vi "AuMT8852B Multiple-slot Sensitivity Configuration.vi"(5 "Settings":T1={"Low frequency selection"=enum."Use low frequency", "Medium frequency selection"=enum."Use medium frequency", "High frequency selection"=enum."Use high frequency", "Low TX frequency"=2480.0, "Low RX frequency"=2402.0, "Medium TX frequency"=2402.0, "Medium RX frequency"=2441.0, "High TX frequency"=2402.0, "High RX frequency"=2480.0, "Number of packets"=590, "TX power"=-70.0, "BER limit"=0.1, "FER limit"=100.0, "Hop selection"=enum."Test with hopping off and on", "Packet type"=enum."Longest supported", "Use Dirty transmitter"=TRUE, "Frequency offset (kHz)"=[71.0, 14.0, -2.0, 1.0, 39.0, 0.0, -42.0, 74.0, -19.0, -75.0], "Modulation index"=[0.33, 0.3, 0.29, 0.32, 0.33, 0.34, 0.29, 0.31, 0.28, 0.35], "Symbol timing error (ppm)"=[-20.0, 20.0, 20.0, 20.0, 20.0, -20.0, -20.0, -20.0, -20.0, 20.0], "Packet count"=enum."RX"} {"Symbol timing error (ppm)" format="%.2f"; "Modulation index" format="%.2f"; "Frequency offset (kHz)" format="%.2f"; "FER limit" format="%.2f"; "BER limit" format="%.2f"; "TX power" format="%.1f"}, 7 "Set/Get (Set)":enum16{"Set", "Get"}(ring), 8 "error in (no error)":errorcluster, 10 "Script (3)":i32=3, 11 "VISA session":refnum<visa-resource-name>) -> (0 "error out":errorcluster, 2 "error code":i32, 3 "VISA session out":refnum<visa-resource-name>, 4 "Settings out":T1={"Low frequency selection"=enum."Use low frequency", "Medium frequency selection"=enum."Use medium frequency", "High frequency selection"=enum."Use high frequency", "Low TX frequency"=0.0, "Low RX frequency"=0.0, "Medium TX frequency"=0.0, "Medium RX frequency"=0.0, "High TX frequency"=0.0, "High RX frequency"=0.0, "Number of packets"=0, "TX power"=0.0, "BER limit"=0.0, "FER limit"=0.0, "Hop selection"=enum."Test with hopping on", "Packet type"=enum."Longest supported", "Use Dirty transmitter"=FALSE, "Frequency offset (kHz)"=[], "Modulation index"=[], "Symbol timing error (ppm)"=[], "Packet count"=enum."TX"} {"Symbol timing error (ppm)" format="%.2f"; "Modulation index" format="%.2f"; "Frequency offset (kHz)" format="%.2f"; "FER limit" format="%.2f"; "BER limit" format="%.2f"; "TX power" format="%.1f"})   [LabVIEW 2017]
doc: "Anritsu MT8852B Bluetooth Tester\n\nConfigures the instrument for the Multiple-slot Sensitivity test.\n\nINPUTS\nSet/Get - whether the values are being sent to or retrieved from the instrument.\nScript - which of the stored scripts (1-10) will be queried or configured. Scripts 1 and 2 are read-only.\nSettings - parameters of the test to be written.\n\nOUTPUTS\nSettings out - current parameters of the test."
uses:
  <instrlib>/aumt8852B/General/Utilities/MT8850 Test Parameters.ctl
  <instrlib>/aumt8852B/General/Utilities/MT8850 Frequency Units.ctl
panel:
  in  "Case Constant\n(See Context Help)":bool
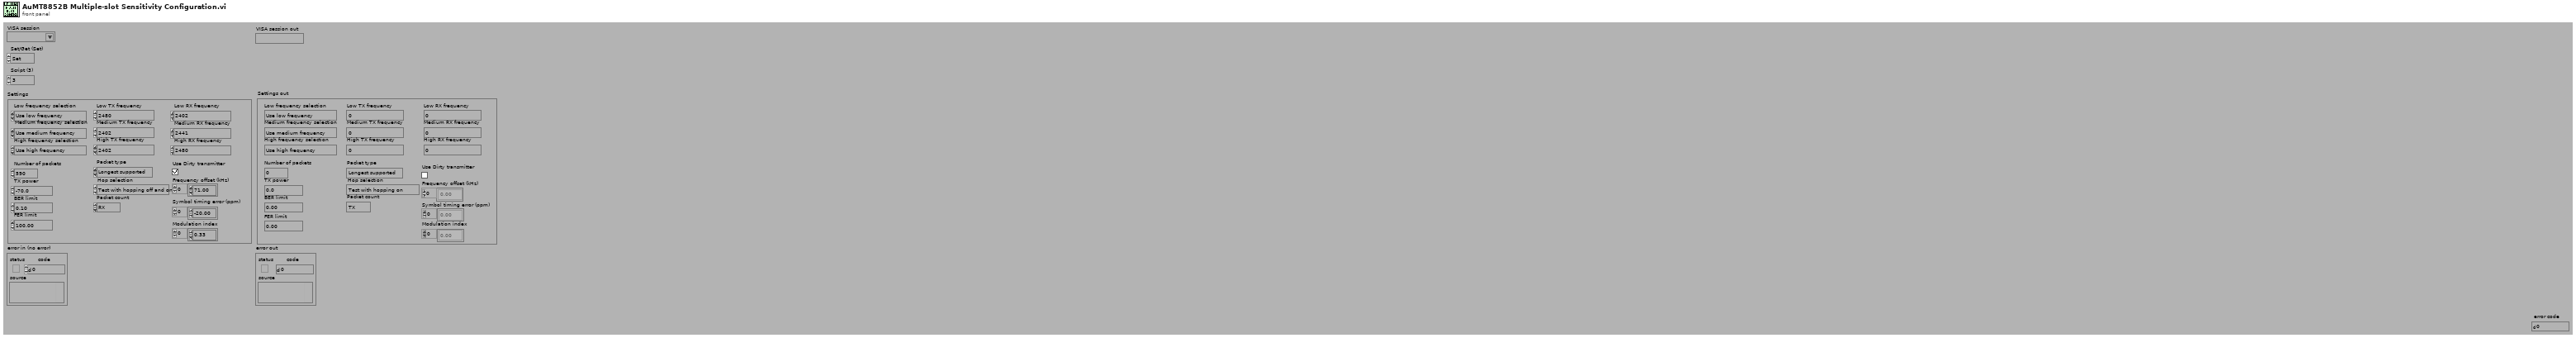
[diagram p1: front panel]
types:
  T1 = cluster{"Low frequency selection":enum16{"Don't use low frequency", "Use low frequency"}, "Medium frequency selection":enum16{"Don't use medium frequency", "Use medium frequency"}, "High frequency selection":enum16{"Don't use high frequency", "Use high frequency"}, "Low TX frequency":dbl, "Low RX frequency":dbl, "Medium TX frequency":dbl, "Medium RX frequency":dbl, "High TX frequency":dbl, "High RX frequency":dbl, "Number of packets":i32, "TX power":dbl, "BER limit":dbl, "FER limit":dbl, "Hop selection":enum16{"Test with hopping on", "Test with hopping off", "Test with hopping off and on"}, "Packet type":enum16{"Longest supported", "DH5", "DH3"}, "Use Dirty transmitter":bool, "Frequency offset (kHz)":dbl[], "Modulation index":dbl[], "Symbol timing error (ppm)":dbl[], "Packet count":enum16{"TX", "RX"}}
  T2 = typedef "MT8850 Test Parameters.ctl" = enum16{"Use low frequency", "Use medium frequency", "Use high frequency", "Low TX frequency", "Low RX frquency", "Medium TX frequency", "Medium RX frequency", "High TX frequency", "High RX frequency", "Number of packets", "Average high limit", "Average low limit", "Peak power limit", "Max power step limit", "Min power step limit", "f1 average minimum", "f1 average maximum", "f2 maximum", "f1/f2 average maximum", "Hop selection", "Use DH1 packets", "Use DH3 packets", "Use DH5 packets", "1 slot packet drift limit", "3 slot packet drift limit", "5 slot packet drift limit", "Drift rate limit", "TX power level", "Frequency offset", "Symbol timing", "Modulation index", "BER limit", "FER limit", "Use averaging high limit", "Use averaging low limit", "Use peak power limit", "Packet type", "Test control", "Use max power step limit", "Use min power step limit", "Number of cycles", "Use f1 average maximum", "Use f1 average minimum", "Use f2 maximum", "Use f1/f2 average maximum", "Hop mode", "Maximum negative limit", "Maximum positive limit", "Use maximum negative limit", "Use maximum positive limit", "Use 1 slot packet drift limit", "Use 3 slot packet drift limit", "Use 5 slot packet drift limit", "Use drift rate limit", "Use BER limit", "Use FER limit", "Use dirty parameter table", "Use null packet drift limit", "Null packet drift limit", "Minimum power", "Power delay", "Packet count", "Payload toggle", "Output power level", "2DHX packet type", "3DHX packet type", "Number of blocks", "TX and RX low frequency", "TX and RX medium frequency", "TX and RX high frequency", "TX frequency", "RX frequency", "Threshold bit count", "Total test bit count", "Number of bits", "PDPSK to PGFSK lower limit", "PDPSK to PGFSK upper limit", "Initial frequency error upper limit", "Initial frequency error lower limit", "Frequency error upper limit", "Frequency error lower limit", "Block frequency error upper limit", "Block frequency error lower limit", "2Mbs RMS DEVM limit", "3Mbs RMS DEVM limit", "2Mbs Peak DEVM limit", "3Mbs Peak DEVM limit", "2Mbs 99% packets DEVM limit", "3Mbs 99% packets DEVM limit", "Percentage of no error packets limit", "Threshold error limit", "Total test error limit"}
  T3 = enum16{"Single-slot sensitivity", "Multiple-slot sensitivity"}
  T4 = enum16{"Frequency offset", "Symbol timing value", "Mod index value"}
  T5 = typedef "MT8850 Frequency Units.ctl" = enum16{"Channel", "Hz", "kHz", "MHz", "GHz"}
  T6 = enum16{"Simulate", "Range check", "Cache", "Query instrument status"}
  T7 = enum16{"Output power", "Power control", "Modulation characteristics", "Initial carrier", "Carrier drift", "Single slot sensitivity", "Multiple slot sensitivity", "Maximum input power"}
  T8 = enum16{"Test with hopping on", "Test with hopping off", "Test with hopping off and on"}
  T9 = enum16{"Don't use high frequency", "Use high frequency"}
  T10 = enum16{"Don't use medium frequency", "Use medium frequency"}
  T11 = enum16{"Don't use low frequency", "Use low frequency"}
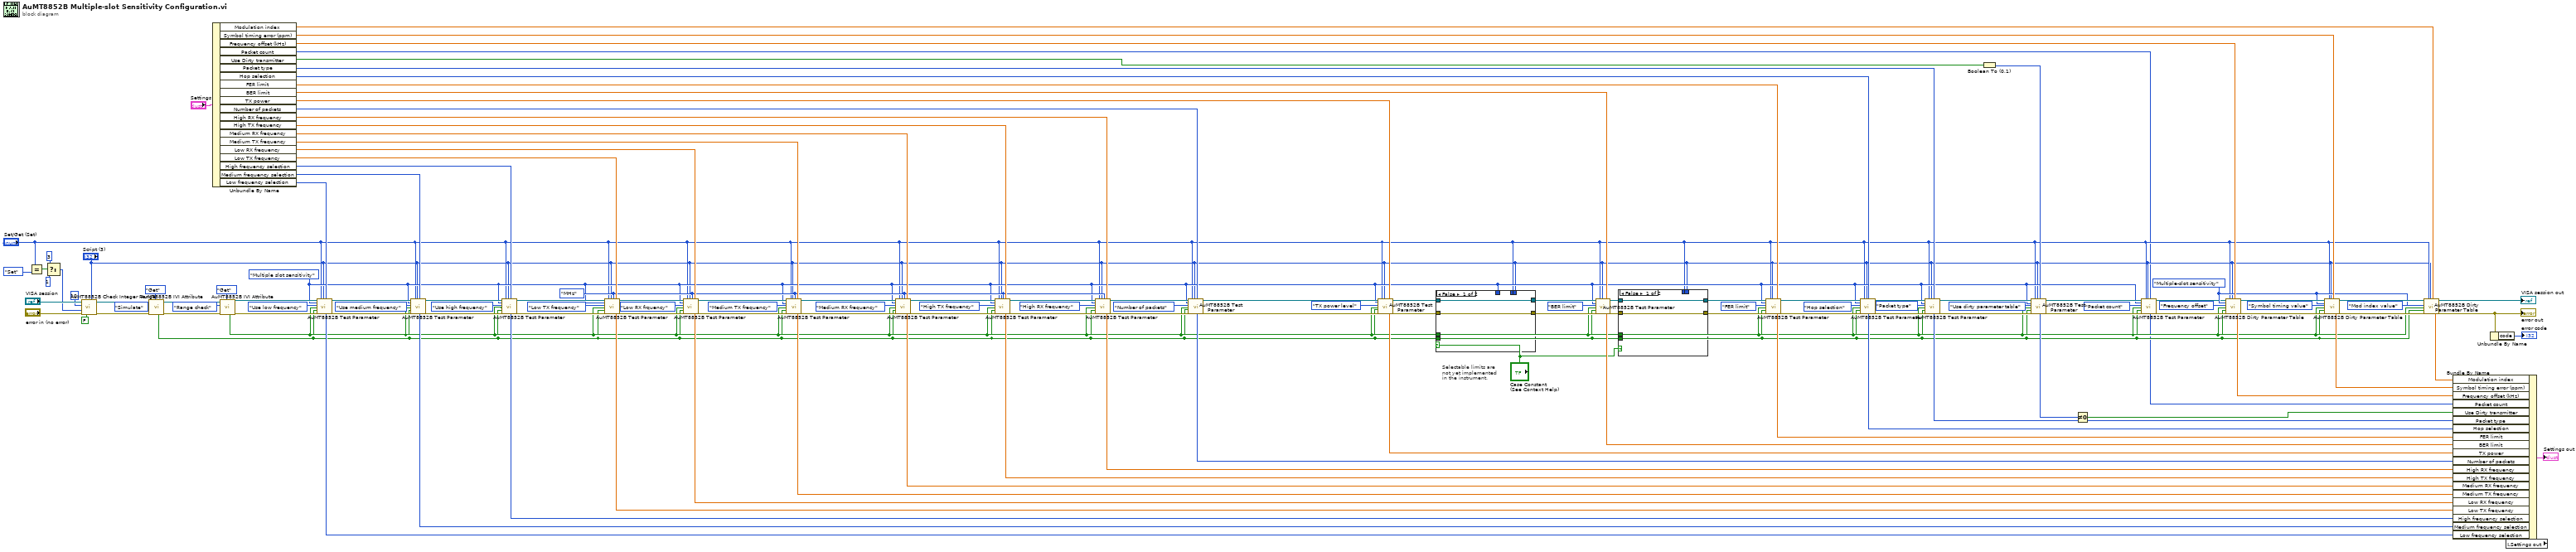
[diagram p0: block diagram]
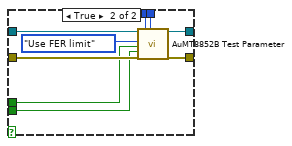
[diagram p2: hidden frame]
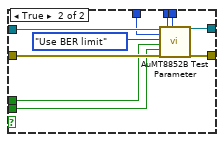
[diagram p3: hidden frame]
diagram:
  w13 = T3."Multiple-slot sensitivity" ("Test (Single-slot sensitivity)")
  w34 = MT8850_Frequency_Units."MHz" ("Frequency units (MHz)")
  w8 = T7."Multiple slot sensitivity" ("Test (Output Power)")
  # "Selectable limits are\nnot yet implemented\nin the instrument."
  n1 = Equal?(x="Set/Get (Set)", y=enum16{"Set", "Get"}."Set") -> (x = y?=w134:bool)
  n2 = Select(t=3, s=w134, f=1) -> (s? t:f=w130:i32)
  n3 = call <instrlib>:"AuMT8852B Check Integer Range.vi"("Value (0)"="Script (3)", "Check IVI flag first? (T)"=FALSE, "error in (no error)"="error in (no error)", "Lower limit (-1)"=w130, "Upper limit (1)"=10, "VISA session"="VISA session") -> ("error out"=w128:errorcluster, "VISA session out"=w129:refnum<visa-resource-name>)  [unwired: 4 in]
  n4 = call <instrlib>:"AuMT8852B IVI Attribute.vi"("Set/Get (Set)"=enum16{"Set", "Get"}."Get", "error in (no error)"=w128, "Flag (Simulate)"=T6."Simulate", "VISA session"=w129) -> ("error out"=w102:errorcluster, "VISA session out"=w103:refnum<visa-resource-name>, "Value out"=w5:bool)  [unwired: 5 in]
  n5 = Unbundle By Name("Settings") -> ("Modulation index"=w23:dbl[], "Symbol timing error (ppm)"=w24:dbl[], "Frequency offset (kHz)"=w28:dbl[], "Packet count"=w1:enum16{"TX", "RX"}, "Use Dirty transmitter"=w46:bool, "Packet type"=w51:enum16{"Longest supported", "DH5", "DH3"}, "Hop selection"=w52:T8, "FER limit"=w70:dbl, "BER limit"=w71:dbl, "TX power"=w75:dbl, "Number of packets"=w76:i32, "High RX frequency"=w89:dbl, "High TX frequency"=w90:dbl, "Medium RX frequency"=w77:dbl, "Medium TX frequency"=w91:dbl, "Low RX frequency"=w92:dbl, "Low TX frequency"=w93:dbl, "High frequency selection"=w94:T9, "Medium frequency selection"=w95:T10, "Low frequency selection"=w96:T11)
  n6 = call <instrlib>:"AuMT8852B IVI Attribute.vi"("Set/Get (Set)"=enum16{"Set", "Get"}."Get", "error in (no error)"=w102, "Flag (Simulate)"=T6."Range check", "VISA session"=w103) -> ("error out"=w100:errorcluster, "VISA session out"=w101:refnum<visa-resource-name>, "Value out"=w6:bool)  [unwired: 5 in]
  n7 = call <instrlib>:"AuMT8852B Test Parameter.vi"("VISA session"=w101, "Test (Output power)"=w8, "Parameter (Use low frequency)"=MT8850_Test_Parameters."Use low frequency", "Range check? (F)"=w6, "Simulate? (F)"=w5, "error in (no error)"=w100, "Set/Get (Set)"="Set/Get (Set)", "Script (3)"="Script (3)", "Integer value (0)"=w96) -> ("Integer value out"=w81:i32, "VISA session out"=w43:refnum<visa-resource-name>, "error out"=w42:errorcluster)  [unwired: 7 in, 1 out]
  n8 = call <instrlib>:"AuMT8852B Test Parameter.vi"("VISA session"=w43, "Test (Output power)"=w8, "Parameter (Use low frequency)"=MT8850_Test_Parameters."Use medium frequency", "Range check? (F)"=w6, "Simulate? (F)"=w5, "error in (no error)"=w42, "Set/Get (Set)"="Set/Get (Set)", "Script (3)"="Script (3)", "Integer value (0)"=w95) -> ("Integer value out"=w82:i32, "VISA session out"=w41:refnum<visa-resource-name>, "error out"=w40:errorcluster)  [unwired: 7 in, 1 out]
  n9 = call <instrlib>:"AuMT8852B Test Parameter.vi"("VISA session"=w41, "Test (Output power)"=w8, "Parameter (Use low frequency)"=MT8850_Test_Parameters."Use high frequency", "Range check? (F)"=w6, "Simulate? (F)"=w5, "error in (no error)"=w40, "Set/Get (Set)"="Set/Get (Set)", "Script (3)"="Script (3)", "Integer value (0)"=w94) -> ("Integer value out"=w83:i32, "VISA session out"=w124:refnum<visa-resource-name>, "error out"=w123:errorcluster)  [unwired: 7 in, 1 out]
  n10 = call <instrlib>:"AuMT8852B Test Parameter.vi"("VISA session"=w124, "Test (Output power)"=w8, "Parameter (Use low frequency)"=MT8850_Test_Parameters."Low TX frequency", "Range check? (F)"=w6, "Simulate? (F)"=w5, "error in (no error)"=w123, "Set/Get (Set)"="Set/Get (Set)", "Script (3)"="Script (3)", "Integer value (0)"=w34, "Float value (0)"=w93) -> ("Float value out"=w84:dbl, "VISA session out"=w122:refnum<visa-resource-name>, "error out"=w121:errorcluster)  [unwired: 6 in, 1 out]
  n11 = call <instrlib>:"AuMT8852B Test Parameter.vi"("VISA session"=w122, "Test (Output power)"=w8, "Parameter (Use low frequency)"=MT8850_Test_Parameters."Low RX frquency", "Range check? (F)"=w6, "Simulate? (F)"=w5, "error in (no error)"=w121, "Set/Get (Set)"="Set/Get (Set)", "Script (3)"="Script (3)", "Integer value (0)"=w34, "Float value (0)"=w92) -> ("Float value out"=w85:dbl, "VISA session out"=w120:refnum<visa-resource-name>, "error out"=w119:errorcluster)  [unwired: 6 in, 1 out]
  n12 = call <instrlib>:"AuMT8852B Test Parameter.vi"("VISA session"=w120, "Test (Output power)"=w8, "Parameter (Use low frequency)"=MT8850_Test_Parameters."Medium TX frequency", "Range check? (F)"=w6, "Simulate? (F)"=w5, "error in (no error)"=w119, "Set/Get (Set)"="Set/Get (Set)", "Script (3)"="Script (3)", "Integer value (0)"=w34, "Float value (0)"=w91) -> ("Float value out"=w86:dbl, "VISA session out"=w118:refnum<visa-resource-name>, "error out"=w117:errorcluster)  [unwired: 6 in, 1 out]
  n13 = call <instrlib>:"AuMT8852B Test Parameter.vi"("VISA session"=w118, "Test (Output power)"=w8, "Parameter (Use low frequency)"=MT8850_Test_Parameters."Medium RX frequency", "Range check? (F)"=w6, "Simulate? (F)"=w5, "error in (no error)"=w117, "Set/Get (Set)"="Set/Get (Set)", "Script (3)"="Script (3)", "Integer value (0)"=w34, "Float value (0)"=w77) -> ("Float value out"=w79:dbl, "VISA session out"=w116:refnum<visa-resource-name>, "error out"=w115:errorcluster)  [unwired: 6 in, 1 out]
  n14 = call <instrlib>:"AuMT8852B Test Parameter.vi"("VISA session"=w116, "Test (Output power)"=w8, "Parameter (Use low frequency)"=MT8850_Test_Parameters."High TX frequency", "Range check? (F)"=w6, "Simulate? (F)"=w5, "error in (no error)"=w115, "Set/Get (Set)"="Set/Get (Set)", "Script (3)"="Script (3)", "Integer value (0)"=w34, "Float value (0)"=w90) -> ("Float value out"=w87:dbl, "VISA session out"=w114:refnum<visa-resource-name>, "error out"=w113:errorcluster)  [unwired: 6 in, 1 out]
  n15 = call <instrlib>:"AuMT8852B Test Parameter.vi"("VISA session"=w114, "Test (Output power)"=w8, "Parameter (Use low frequency)"=MT8850_Test_Parameters."High RX frequency", "Range check? (F)"=w6, "Simulate? (F)"=w5, "error in (no error)"=w113, "Set/Get (Set)"="Set/Get (Set)", "Script (3)"="Script (3)", "Integer value (0)"=w34, "Float value (0)"=w89) -> ("Float value out"=w88:dbl, "VISA session out"=w112:refnum<visa-resource-name>, "error out"=w111:errorcluster)  [unwired: 6 in, 1 out]
  n16 = call <instrlib>:"AuMT8852B Test Parameter.vi"("VISA session"=w112, "Test (Output power)"=w8, "Parameter (Use low frequency)"=MT8850_Test_Parameters."Number of packets", "Range check? (F)"=w6, "Simulate? (F)"=w5, "error in (no error)"=w111, "Set/Get (Set)"="Set/Get (Set)", "Script (3)"="Script (3)", "Integer value (0)"=w76) -> ("Integer value out"=w78:i32, "VISA session out"=w31:refnum<visa-resource-name>, "error out"=w30:errorcluster)  [unwired: 7 in, 1 out]
  n17 = call <instrlib>:"AuMT8852B Test Parameter.vi"("VISA session"=w31, "Test (Output power)"=w8, "Parameter (Use low frequency)"=MT8850_Test_Parameters."TX power level", "Range check? (F)"=w6, "Simulate? (F)"=w5, "error in (no error)"=w30, "Set/Get (Set)"="Set/Get (Set)", "Script (3)"="Script (3)", "Float value (0)"=w75) -> ("Float value out"=w69:dbl, "VISA session out"=w26:refnum<visa-resource-name>, "error out"=w27:errorcluster)  [unwired: 7 in, 1 out]
  n18 = case shown="False" "Case Constant\n(See Context Help)" {
    tunnel: w27 -> [w138 w148]
    tunnel: w26 -> [w139 w147]
    tunnel: [w139 w146] -> w58
    tunnel: [w138 w145] -> w57
    tunnel: w6 -> [_ w144]
    tunnel: w5 -> [_ w143]
    tunnel: w8 -> [_ w142]
    tunnel: "Set/Get (Set)" -> [_ w141]
    tunnel: "Script (3)" -> [_ w140]
    frame False {
    }
    frame True {
      n19 = call <instrlib>:"AuMT8852B Test Parameter.vi"("VISA session"=w147, "Test (Output power)"=w142, "Parameter (Use low frequency)"=MT8850_Test_Parameters."Use BER limit", "Range check? (F)"=w144, "Simulate? (F)"=w143, "error in (no error)"=w148, "Set/Get (Set)"=w141, "Script (3)"=w140) -> ("VISA session out"=w146:refnum<visa-resource-name>, "error out"=w145:errorcluster)  [unwired: 8 in, 2 out]
    }
  }
  n20 = call <instrlib>:"AuMT8852B Test Parameter.vi"("VISA session"=w58, "Test (Output power)"=w8, "Parameter (Use low frequency)"=MT8850_Test_Parameters."BER limit", "Range check? (F)"=w6, "Simulate? (F)"=w5, "error in (no error)"=w57, "Set/Get (Set)"="Set/Get (Set)", "Script (3)"="Script (3)", "Float value (0)"=w71) -> ("Float value out"=w68:dbl, "VISA session out"=w55:refnum<visa-resource-name>, "error out"=w56:errorcluster)  [unwired: 7 in, 1 out]
  n21 = case shown="False" "Case Constant\n(See Context Help)" {
    tunnel: w56 -> [w150 w159]
    tunnel: w55 -> [w151 w158]
    tunnel: [w151 w157] -> w54
    tunnel: [w150 w156] -> w53
    tunnel: w6 -> [_ w155]
    tunnel: w5 -> [_ w154]
    tunnel: "Set/Get (Set)" -> [_ w153]
    tunnel: "Script (3)" -> [_ w152]
    frame False {
    }
    frame True {
      n22 = call <instrlib>:"AuMT8852B Test Parameter.vi"("VISA session"=w158, "Parameter (Use low frequency)"=MT8850_Test_Parameters."Use FER limit", "Range check? (F)"=w155, "Simulate? (F)"=w154, "error in (no error)"=w159, "Set/Get (Set)"=w153, "Script (3)"=w152) -> ("VISA session out"=w157:refnum<visa-resource-name>, "error out"=w156:errorcluster)  [unwired: 9 in, 2 out]
    }
  }
  n23 = call <instrlib>:"AuMT8852B Test Parameter.vi"("VISA session"=w54, "Test (Output power)"=w8, "Parameter (Use low frequency)"=MT8850_Test_Parameters."FER limit", "Range check? (F)"=w6, "Simulate? (F)"=w5, "error in (no error)"=w53, "Set/Get (Set)"="Set/Get (Set)", "Script (3)"="Script (3)", "Float value (0)"=w70) -> ("Float value out"=w67:dbl, "VISA session out"=w61:refnum<visa-resource-name>, "error out"=w64:errorcluster)  [unwired: 7 in, 1 out]
  n24 = call <instrlib>:"AuMT8852B Test Parameter.vi"("VISA session"=w61, "Test (Output power)"=w8, "Parameter (Use low frequency)"=MT8850_Test_Parameters."Hop selection", "Range check? (F)"=w6, "Simulate? (F)"=w5, "error in (no error)"=w64, "Set/Get (Set)"="Set/Get (Set)", "Script (3)"="Script (3)", "Integer value (0)"=w52) -> ("Integer value out"=w60:i32, "VISA session out"=w62:refnum<visa-resource-name>, "error out"=w63:errorcluster)  [unwired: 7 in, 1 out]
  n25 = call <instrlib>:"AuMT8852B Test Parameter.vi"("VISA session"=w62, "Test (Output power)"=w8, "Parameter (Use low frequency)"=MT8850_Test_Parameters."Packet type", "Range check? (F)"=w6, "Simulate? (F)"=w5, "error in (no error)"=w63, "Set/Get (Set)"="Set/Get (Set)", "Script (3)"="Script (3)", "Integer value (0)"=w51) -> ("Integer value out"=w59:i32, "VISA session out"=w32:refnum<visa-resource-name>, "error out"=w33:errorcluster)  [unwired: 7 in, 1 out]
  n26 = Boolean To (0,1)(Boolean=w46) -> (0, 1=w47:i16)
  n27 = call <instrlib>:"AuMT8852B Test Parameter.vi"("VISA session"=w32, "Test (Output power)"=w8, "Parameter (Use low frequency)"=MT8850_Test_Parameters."Use dirty parameter table", "Range check? (F)"=w6, "Simulate? (F)"=w5, "error in (no error)"=w33, "Set/Get (Set)"="Set/Get (Set)", "Script (3)"="Script (3)", "Integer value (0)"=w47) -> ("Integer value out"=w48:i32, "VISA session out"=w12:refnum<visa-resource-name>, "error out"=w11:errorcluster)  [unwired: 7 in, 1 out]
  n28 = Not Equal To 0?(x=w48) -> (x != 0?=w49:bool)
  n29 = call <instrlib>:"AuMT8852B Test Parameter.vi"("VISA session"=w12, "Test (Output power)"=w8, "Parameter (Use low frequency)"=MT8850_Test_Parameters."Packet count", "Range check? (F)"=w6, "Simulate? (F)"=w5, "error in (no error)"=w11, "Set/Get (Set)"="Set/Get (Set)", "Script (3)"="Script (3)", "Integer value (0)"=w1) -> ("Integer value out"=w2:i32, "VISA session out"=w9:refnum<visa-resource-name>, "error out"=w10:errorcluster)  [unwired: 7 in, 1 out]
  n30 = call <instrlib>:"AuMT8852B Dirty Parameter Table.vi"("VISA session"=w9, "Test (Single-slot sensitivity)"=w13, "Variable (Frequency offset)"=T4."Frequency offset", "Range check? (F)"=w6, "Simulate? (F)"=w5, "error in (no error)"=w10, "Set/Get (Set)"="Set/Get (Set)", "Script (3)"="Script (3)", "Parameters"=w28) -> ("Parameters out"=w29:dbl[], "VISA session out"=w19:refnum<visa-resource-name>, "error out"=w18:errorcluster)  [unwired: 8 in]
  n31 = call <instrlib>:"AuMT8852B Dirty Parameter Table.vi"("VISA session"=w19, "Test (Single-slot sensitivity)"=w13, "Variable (Frequency offset)"=T4."Symbol timing value", "Range check? (F)"=w6, "Simulate? (F)"=w5, "error in (no error)"=w18, "Set/Get (Set)"="Set/Get (Set)", "Script (3)"="Script (3)", "Parameters"=w24) -> ("Parameters out"=w25:dbl[], "VISA session out"=w16:refnum<visa-resource-name>, "error out"=w15:errorcluster)  [unwired: 8 in]
  n32 = call <instrlib>:"AuMT8852B Dirty Parameter Table.vi"("VISA session"=w16, "Test (Single-slot sensitivity)"=w13, "Variable (Frequency offset)"=T4."Mod index value", "Range check? (F)"=w6, "Simulate? (F)"=w5, "error in (no error)"=w15, "Set/Get (Set)"="Set/Get (Set)", "Script (3)"="Script (3)", "Parameters"=w23) -> ("Parameters out"=w22:dbl[], "VISA session out"=→"VISA session out":refnum<visa-resource-name>, "error out"=w36:errorcluster)  [unwired: 8 in]
  "error out" <- w36
  n33 = Unbundle By Name(w36) -> ("code"=→"error code":i32)
  n34 = local read "Settings out"() -> (w80:T1)
  n35 = Bundle By Name(cluster=w80, "Modulation index"=w22, "Symbol timing error (ppm)"=w25, "Frequency offset (kHz)"=w29, "Packet count"=w2, "Use Dirty transmitter"=w49, "Packet type"=w59, "Hop selection"=w60, "FER limit"=w67, "BER limit"=w68, "TX power"=w69, "Number of packets"=w78, "High RX frequency"=w88, "High TX frequency"=w87, "Medium RX frequency"=w79, "Medium TX frequency"=w86, "Low RX frequency"=w85, "Low TX frequency"=w84, "High frequency selection"=w83, "Medium frequency selection"=w82, "Low frequency selection"=w81) -> (→"Settings out":T1)
